vi "Send Initiallize EMG Task.vi"(5 "TDMS File":refnum<k34>, 7 "Priority":T2=enum."Normal" caption="Message Priority (Normal)", 8 "error in (no error)":errorcluster, 9 "EMG Master Config":T1, 10 "EMG info":cluster{"Collect EMG?":bool, "EMG Rate":u16}, 11 "Message Enqueuer in":refnum<class "Message Enqueuer.lvclass">) -> (0 "error out":errorcluster, 3 "Message Enqueuer out":refnum<class "Message Enqueuer.lvclass">)   [LabVIEW 2020, in "NI Force Task.lvlib" / "Initiallize EMG Task Msg.lvclass"]
doc: "Sends the <b>NI Force Task.lvlib:Initiallize EMG Task Msg.lvclass</b> message.\n\nThis message will call <b>Initiallize EMG Task.vi</b> on the <b>NI Force Task.lvlib:NI Force Task.lvclass</b> actor.\n\n<b>Initiallize EMG Task.vi Description</b>"
uses:
  Initiallize EMG Task Msg.lvclass
  <vilib>/ActorFramework/Message Enqueuer/Message Enqueuer.lvclass
  <vilib>/ActorFramework/Message Enqueuer/Message Priority.ctl
  EMG channels df.ctl
  C:/Program Files/National Instruments/LabVIEW 2020/vi.lib/ActorFramework/Message/Message.lvclass
  Initiallize EMG Task Msg.lvclass/Initiallize EMG Task Msg.ctl
  <vilib>/ActorFramework/Message Enqueuer/Message Enqueuer.lvclass/Message Enqueuer.ctl
  <vilib>/ActorFramework/Message Priority Queue/Priority Enqueue.vi
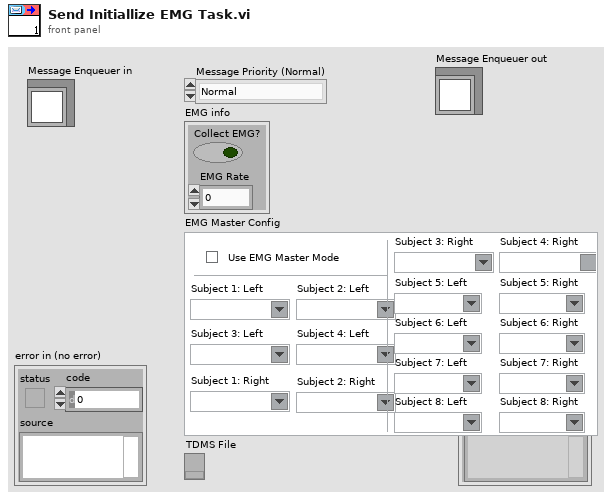
[diagram p1: front panel]
types:
  T1 = typedef "EMG channels df.ctl" = cluster{"EMG Master":bool, "EMGL1":tag, "EMGR1":tag, "EMGL2":tag, "EMGR2":tag, "EMGL3":tag, "EMGR3":tag, "EMGL4":tag, "EMGR4":tag, "EMGL5":tag, "EMGR5":tag, "EMGL6":tag, "EMGR6":tag, "EMGL7":tag, "EMGR7":tag, "EMGL8":tag, "EMGR8":tag}
  T2 = typedef "Actor Framework.lvlib/Message Enqueuer.lvclass/Message Priority.ctl" = enum16{"Low", "Normal", "High"}
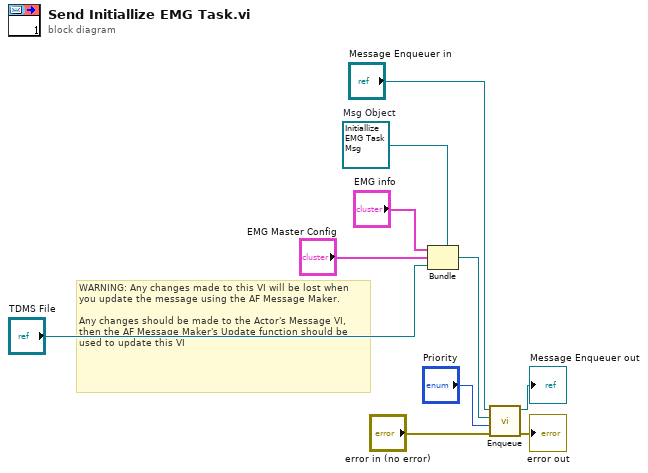
[diagram p0: block diagram]
diagram:
  w7 = refnum<class "Initiallize EMG Task Msg.lvclass"> refnum  # Msg Object
  # "WARNING: Any changes made to this VI will be lost when you update the message using the AF Message Maker.\n\nAny changes should be made to the Actor's Message VI, then the AF Message Maker's Update function should be used to update this VI"
  n1 = Bundle(cluster=w7, "EMG info", "EMG Master Config", "TDMS File") -> (w2:refnum<class "Initiallize EMG Task Msg.lvclass">)
  n2 = call <vilib>:"Enqueue.vi"("error in (no error)"="error in (no error)", "Message Priority (Normal)"="Priority", "Message"=w2, "Message Enqueuer in"="Message Enqueuer in") -> ("error out"=→"error out":errorcluster, "Message Enqueuer out"=→"Message Enqueuer out":refnum<class "Message Enqueuer.lvclass">)  [unwired: 6 in]
